vi "Insight_R_Invalid_Data_Indices.vi"(8 "error in (no error)":errorcluster, 11 "telnet connection":T1) -> (0 "error out":errorcluster, 1 "response data":string, 2 "Invalid Data Indices":i32[](array[numeric]), 3 "telnet  connection out":T1)   [LabVIEW 2015]
doc: "Insight Photonic Solutions\n\nThis VI reads the Indices of the Invalid Data in the sweep.\n\nver 2.0 - updated command syntax\nver 2.1 - return the full response string\nver 3.3 - parses response for Atlas 3.3 and newer, and Atlas 3.2 and earlier\nver 4.3 - updated Scan from String to handle new DIV format in Atlas 4.3"
uses:
  Telnet Session.ctl
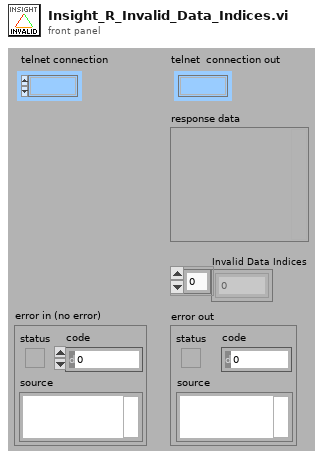
[diagram p1: front panel]
types:
  T1 = typedef "Telnet Session.ctl" = refnum<k1>
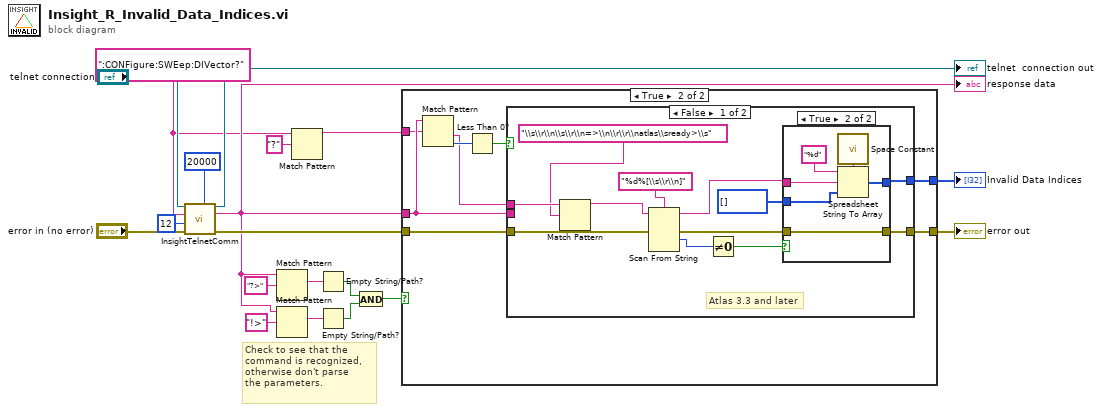
[diagram p0: block diagram]
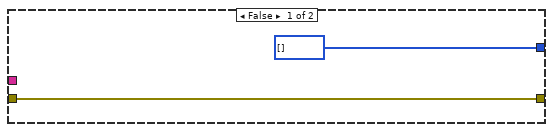
[diagram p2: hidden frame]
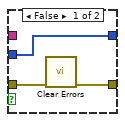
[diagram p3: hidden frame]
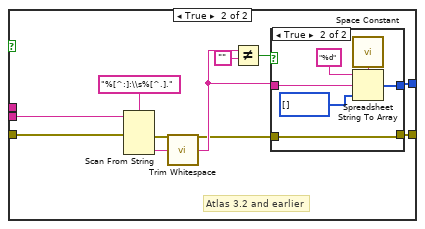
[diagram p4: hidden frame]
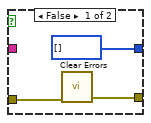
[diagram p5: hidden frame]
diagram:
  w2 = ":CONFigure:SWEep:DIVector?" ("String")
  # "Check to see that the \ncommand is recognized,\notherwise don't parse \nthe parameters."
  n1 = call "InsightTelnetComm.vi"("bytes to read"=20000, "error in"="error in (no error)", "Timeout, sec"=u32 12, "write buffer (\"\")"=w2, "telnet connection"="telnet connection") -> ("error out"=w15:errorcluster, "response data"=w5:string, "telnet  connection out"=→"telnet  connection out":T1)  [unwired: 2 in]
  "response data" <- w5
  n2 = Match Pattern(string=w5, regular expression="?>") -> (match substring=w7:string)  [unwired: 1 in, 3 out]
  n3 = Match Pattern(string=w5, regular expression="!>") -> (match substring=w8:string)  [unwired: 1 in, 3 out]
  n4 = Match Pattern(string=w2, regular expression="?") -> (before substring=w1:string)  [unwired: 1 in, 3 out]
  n5 = Empty String/Path?(string/path=w7) -> (empty?=w10:bool)
  n6 = Empty String/Path?(string/path=w8) -> (empty?=w11:bool)
  n7 = And(x=w10, y=w11) -> (x .and. y?=w4:bool)
  n8 = case shown="True" w4 {
    tunnel: [i32[] [] w29] -> w16
    tunnel: w15 -> [w20 w28]
    tunnel: [w20 w27] -> w13
    tunnel: w5 -> [_ w26]
    tunnel: w1 -> [_ w25]
    frame False {
    }
    frame True {
      n9 = Match Pattern(string=w26, regular expression=w25) -> (after substring=w22:string, offset past match=w24:i32)  [unwired: 1 in, 2 out]
      n10 = Less Than 0?(x=w24) -> (x < 0?=w23:bool)
      n11 = case shown="False" w23 {
        tunnel: [w38 w60] -> w29
        tunnel: w28 -> [w40 w58]
        tunnel: [w33 w54] -> w27
        tunnel: w26 -> [_ w51]
        tunnel: w22 -> [w32 _]
        frame False {
          # "Atlas 3.3 and later"
          n12 = Match Pattern(string=w32, regular expression="\\s\\r\\n\\s\\r\\n=>\\n\\r\\r\\natlas\\sready>\\s" ("format string")) -> (before substring=w30:string)  [unwired: 1 in, 3 out]
          n13 = Scan From String(format string="%d%[\\s\\r\\n]", input string=w30, error in=w40) -> (remaining string=w37:string, error out=w34:errorcluster, output 1=w36:i32)  [unwired: 4 in, 1 out]
          n14 = Not Equal To 0?(x=w36) -> (x != 0?=w35:bool)
          n15 = case shown="True" w35 {
            tunnel: i32[] [] -> [w44 w49]
            tunnel: [w44 w47] -> w38
            tunnel: w37 -> [_ w46]
            tunnel: w34 -> [w43 w45]
            tunnel: [w42 w45] -> w33
            frame False {
              n16 = call <vilib>:"Clear Errors.vi"("error in (no error)"=w43) -> ("error out"=w42:errorcluster)  [unwired: 5 in, 1 out]
            }
            frame True {
              n17 = call <vilib>:"Space Constant.vi"() -> ("String"=w48:string)
              n18 = Spreadsheet String To Array(delimiter (Tab)=w48, format string="%d", spreadsheet string=w46, array type (2D Dbl)=w49) -> (array=w47:i32[])
            }
          }
        }
        frame True {
          # "Atlas 3.2 and earlier"
          n19 = Scan From String(format string="%[^:]:\\s%[^.].", input string=w51, error in=w58) -> (error out=w53:errorcluster, output 2=w52:string)  [unwired: 4 in, 2 out]
          n20 = call <vilib>:"Trim Whitespace.vi"("string"=w52) -> ("trimmed string"=w56:string)  [unwired: 1 in]
          n21 = Not Equal?(x=w56, y="") -> (x != y?=w55:bool)
          n22 = case shown="True" w55 {
            tunnel: [i32[] [] w66] -> w60
            tunnel: w56 -> [_ w65]
            tunnel: [w63 w64] -> w54
            tunnel: w53 -> [w62 w64]
            frame False {
              n23 = call <vilib>:"Clear Errors.vi"("error in (no error)"=w62) -> ("error out"=w63:errorcluster)  [unwired: 5 in, 1 out]
            }
            frame True {
              n24 = call <vilib>:"Space Constant.vi"() -> ("String"=w67:string)
              n25 = Spreadsheet String To Array(delimiter (Tab)=w67, format string="%d", spreadsheet string=w65, array type (2D Dbl)=i32[] []) -> (array=w66:i32[])
            }
          }
        }
      }
    }
  }
  "error out" <- w13
  "Invalid Data Indices" <- w16
